vi "Listening Server - Initialize.vi"(8 "error in (no error)":errorcluster, 11 "Plugin in":refnum<class "Generic Plugin.lvclass">) -> (0 "error out":errorcluster, 2 "Listening Server Reference":refnum<vi>, 3 "Plugin out":refnum<class "Generic Plugin.lvclass">)   [LabVIEW 2020, in "RxnRover.lvlib" / "Generic Plugin.lvclass"]
uses:
  Generic Plugin.lvclass
  Generic Plugin.lvclass/Generic Plugin.ctl
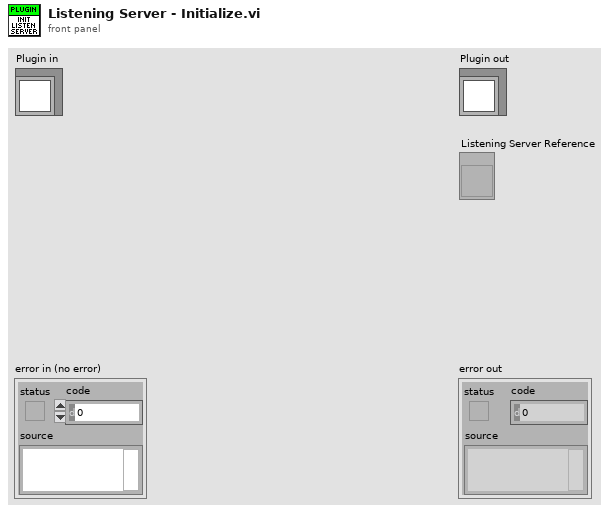
[diagram p1: front panel]
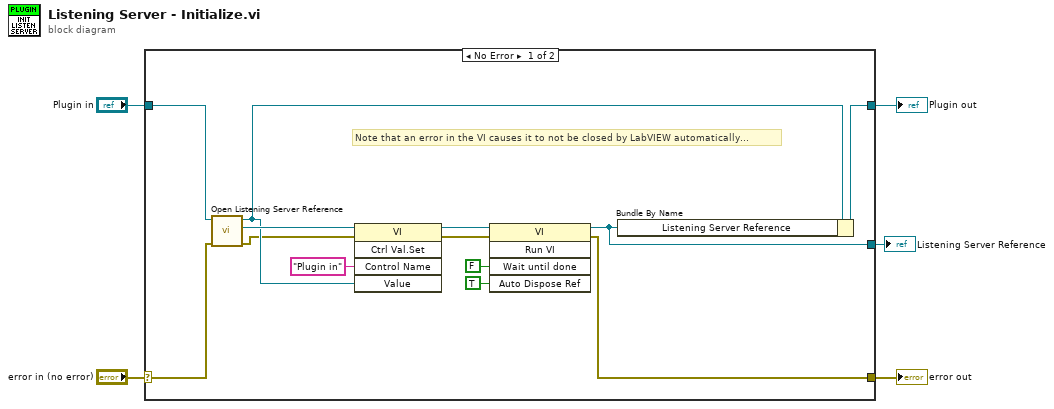
[diagram p0: block diagram]
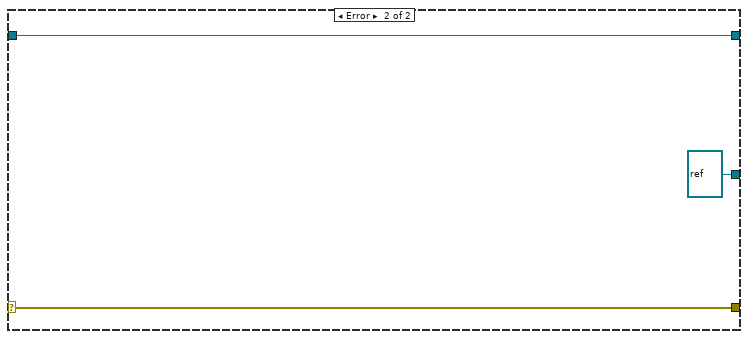
[diagram p2: hidden frame]
diagram:
  n1 = case shown="No Error" "error in (no error)" {
    selector: "error in (no error)" -> [w17 w21]
    tunnel: [w8 w21] -> w4
    tunnel: [w7 w20] -> w2
    tunnel: "Plugin in" -> [w18 w20]
    tunnel: [w6 refnum<vi> refnum ("vi reference")] -> w1
    frame No Error {
      # "Note that an error in the VI causes it to not be closed by LabVIEW automatically..."
      n2 = call-dynamic "Open Listening Server Reference.vi"("error in (no error)"=w17, "Plugin in"=w18) -> ("error out"=w13:errorcluster, "vi reference"=w16:refnum<vi>, "Plugin out"=w14:refnum<class "Generic Plugin.lvclass">)  [unwired: 7 in]
      n3 = invoke class="VI" method="Ctrl Val.Set"(reference=w16, error in=w13, "Control Name"="Plugin in", "Value"=w14) -> (reference out=w12:refnum<vi>, error out=w11:errorcluster)  [unwired: 1 in, 3 out]
      n4 = invoke class="VI" method="Run VI"(reference=w12, error in=w11, "Wait until done"=FALSE ("Wait Until Done"), "Auto Dispose Ref"=TRUE ("Auto Dispose Reference")) -> (reference out=w6:refnum<vi>, error out=w8:errorcluster)  [unwired: 1 in, 3 out]
      n5 = Bundle By Name(cluster=w14, "Listening Server Reference"=w6) -> (w7:refnum<class "Generic Plugin.lvclass">)
    }
    frame Error {
    }
  }
  "error out" <- w4
  "Plugin out" <- w2
  "Listening Server Reference" <- w1
